vi "Manual with gyro correction - fun no timed loop.vi"() -> ()   [LabVIEW 2017]
panel:
  in  "Encoder Scale":dbl=6.55
  out "y out":dbl format="%#.6f"
  out "x out":dbl format="%#.6f"
  out "Rot spd out":dbl
  out "Remaining delay":dbl
  in  "Period":i64=10
  in  "Delay (s)":dbl
  in  "Motor Stop":bool
  in  "Anticlockwise":bool
  in  "Clockwise":bool
  out "Command from keys":T1(ring)
  in  "Right":bool
  in  "Left":bool
  in  "Down":bool
  in  "Up":bool
  in  "Rot spd multiplier":dbl=2.0
  out "motor 2 out":dbl format="%#.4f"
  out "motor 4 out":dbl format="%#.4f"
  out "motor 3 out":dbl format="%#.4f"
  out "motor 1 out":dbl format="%#.4f"
  out "error out":errorcluster
  in  "error in":errorcluster
  in  "Trans speed":dbl=3.0
  out "Speed C0":T2(graph)
  out "Counter C0":i32
  out "dx/dt C0":dbl
  out "Speed A":T2(graph)
  out "Counter B":i32
  out "Speed B":T2(graph)
  out "dx/dt B":dbl
  out "dt out (s)":dbl format="%.3f"
  in  "PID gains":T3={"proportional gain (Kc)"=0.015, "integral time (Ti, min)"=0.003, "derivative time (Td, min)"=0.0} {"derivative time (Td, min)" format="%.6f"; "integral time (Ti, min)" format="%.6f"; "proportional gain (Kc)" format="%.6f"}
  in  "stop":bool
  out "dx/dt A":dbl
  out "Counter A":i32
  # "P:  Higher the number, higher the abrupt change\nI: Higher the number, the less it tries to overshoot"
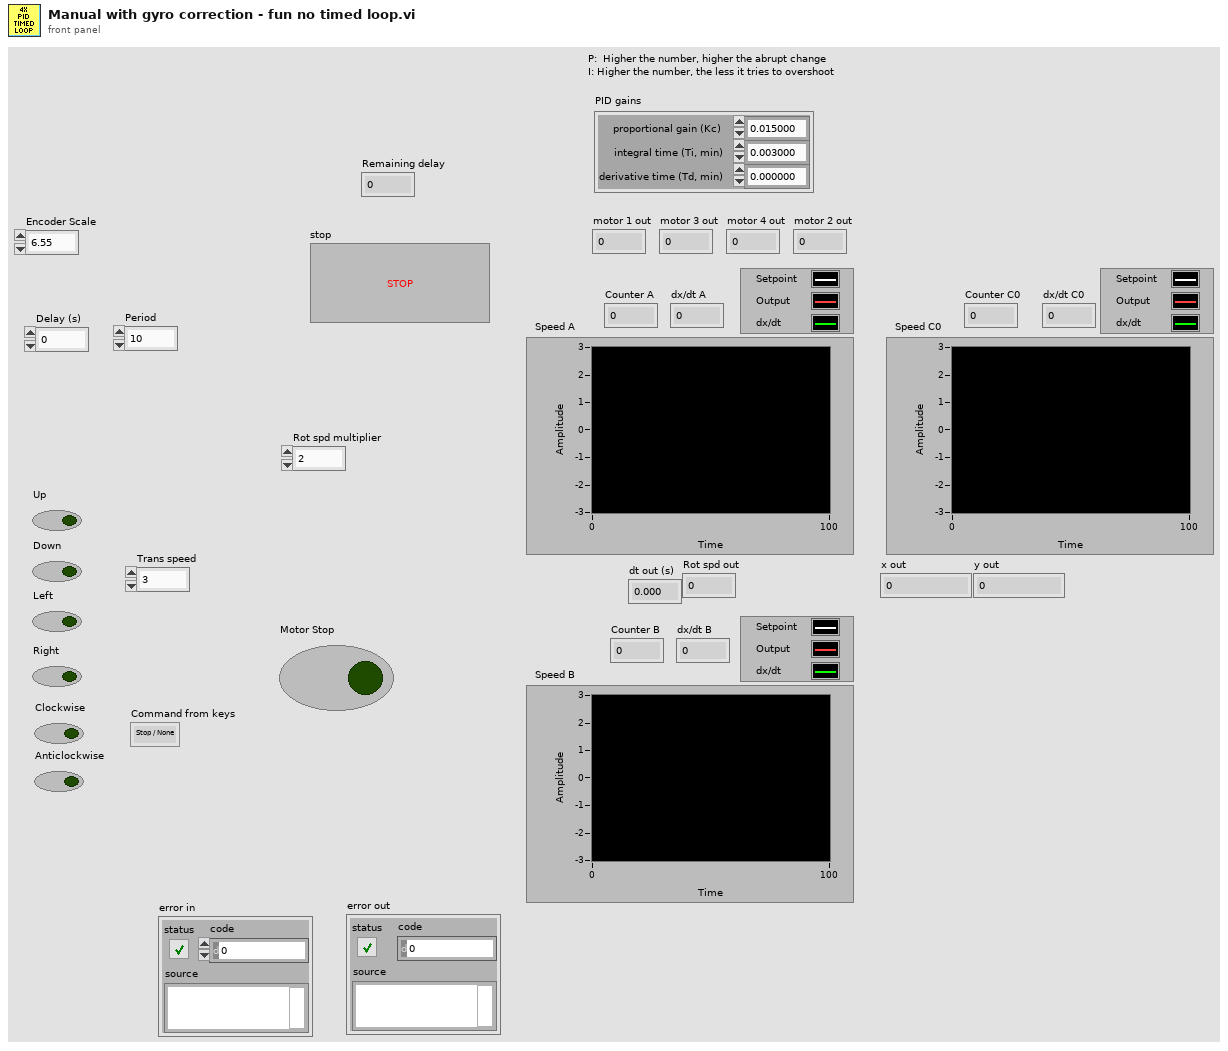
[diagram p1: front panel]
types:
  T1 = enum16{"Stop / None", "Forward", "Backward", "Left", "Right", "Manual"}
  T2 = cluster{"Setpoint":dbl, "output":dbl, "dx/dt":dbl}
  T3 = cluster{"proportional gain (Kc)":dbl, "integral time (Ti, min)":dbl, "derivative time (Td, min)":dbl}
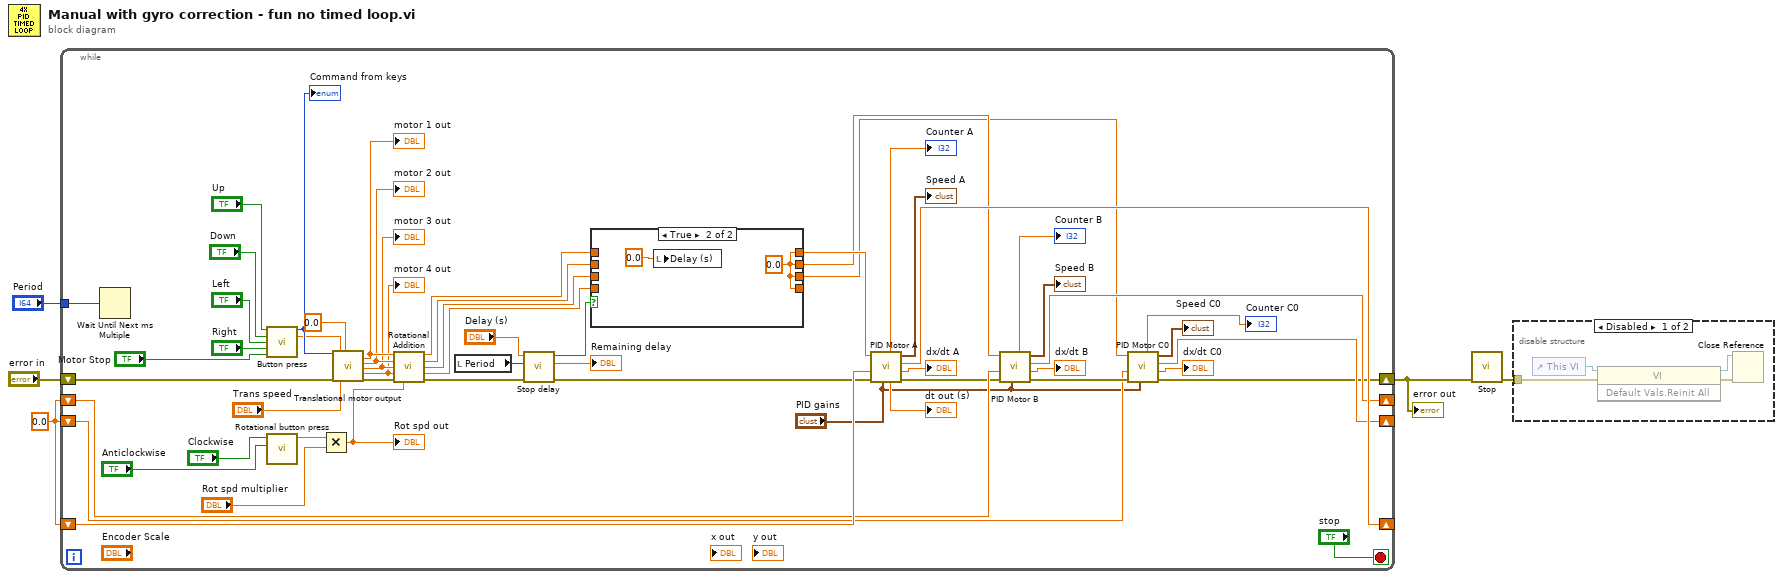
[diagram p0: block diagram]
diagram:
  w5 = 0.0 ("output")
  n1 = while {
    shift-right: [w56] -> _
    shift-left: w5 -> [w60]
    shift-right: [w55] -> _
    shift-left: w5 -> [w54]
    shift-right: [w51] -> _
    shift-left: w5 -> [w50]
    shift-right: [w6] -> w2
    shift-left: "error in" -> [w29]
    tunnel: "Period" -> [w13]
    stop <- "stop" stop-if-true
    n2 = Wait Until Next ms Multiple(millisecond multiple=w13) -> ()  [unwired: 1 out]
    n3 = call "Button press.vi"("Up"="Up", "Down"="Down", "Left"="Left", "Right"="Right", "Stop"="Motor Stop") -> ("Command"=w37:T1, "angle"=w31:dbl)  [unwired: 9 in]
    "Command from keys" <- w37
    n4 = call "Rotational button press.vi"("Anticlockwise"="Anticlockwise", "Clockwise"="Clockwise") -> ("rotDirection"=w7:dbl)  [unwired: 9 in]
    n5 = Multiply(x=w7, y="Rot spd multiplier") -> (x*y=w28:dbl)
    "Rot spd out" <- w28
    n6 = call "Translational motor output.vi"("Command"=w37, "error in"=w29, "manual input angle"=w31, "Trans spd multiplier"="Trans speed", "Orientation"=0.0 ("integral processed")) -> ("motor 1 out"=w43:dbl, "motor 2 out"=w42:dbl, "motor 3 out"=w41:dbl, "motor 4 out"=w40:dbl, "error out"=w39:errorcluster)  [unwired: 10 in]
    "motor 1 out" <- w43
    "motor 3 out" <- w41
    "motor 4 out" <- w40
    "motor 2 out" <- w42
    n7 = call "Rotational Addition.vi"("Motor 1 in"=w43, "Motor 2 in"=w42, "Motor 3 in"=w41, "Motor 4 in"=w40, "error in"=w39, "Rot spd multiplier"=w28) -> ("Motor 1 out"=w27:dbl, "Motor 2 out"=w25:dbl, "Motor 3 out"=w23:dbl, "Motor 4 out"=w21:dbl, "error out"=w20:errorcluster)  [unwired: 5 in]
    n8 = local read "Period"() -> (w16:i64)
    n9 = call "Stop delay.vi"("error in (no error)"=w20, "Period (ms)"=w16, "Delay (s)"="Delay (s)") -> ("error out"=w19:errorcluster, "Remaining delay"=→"Remaining delay":dbl, "Stop?"=w18:bool)  [unwired: 6 in]
    n10 = case shown="True" w18 {
      tunnel: w27 -> [w61 _]
      tunnel: [w61 w66] -> w26
      tunnel: w25 -> [w64 _]
      tunnel: [w64 w66] -> w24
      tunnel: w23 -> [w63 _]
      tunnel: [w63 w66] -> w22
      tunnel: w21 -> [w62 _]
      tunnel: [w62 w66] -> _
      frame False {
      }
      frame True {
        w66 = 0.0 ("Motor 4 out")
        n11 = local write "Delay (s)"(0.0 ("Delay (s)")) -> ()
      }
    }
    n12 = call "PID Motor A.vi"("PID gains"="PID gains", "error in (no error)"=w19, "input"=w60, "Setpoint A0"=w26) -> ("error out"=w45:errorcluster, "dx/dt processed"=→"dx/dt A":dbl, "output"=w56:dbl, "Speed A0"=→"Speed A":T2, "dt out (s)"=→"dt out (s)":dbl, "Counter A0"=→"Counter A":dbl)  [unwired: 2 in]
    n13 = call "PID Motor B.vi"("PID gains"="PID gains", "error in (no error)"=w45, "input"=w54, "Setpoint B0"=w24) -> ("error out"=w52:errorcluster, "dx/dt"=→"dx/dt B":dbl, "output"=w55:dbl, "Speed B0"=→"Speed B":T2, "Counter B0"=→"Counter B":dbl)  [unwired: 2 in, 1 out]
    n14 = call "PID Motor C0.vi"("PID gains"="PID gains", "error in (no error)"=w52, "input"=w50, "Setpoint C0"=w22) -> ("error out"=w6:errorcluster, "dx/dt"=→"dx/dt C0":dbl, "output"=w51:dbl, "Speed C0"=→"Speed C0":T2, "Counter C0"=→"Counter C0":dbl)  [unwired: 2 in, 1 out]
  }
  "error out" <- w2
  n15 = call "Stop.vi"("error in (no error)"=w2) -> ("OG error out"=w3:errorcluster)  [unwired: 9 in, 1 out]
  n16 = disable-structure shown="Disabled" {
    disable-tunnel: w3 -> [w70 _]
    frame Disabled {
      n17 = control-ref of="This VI"() -> (w69:refnum<vi>)
      n18 = invoke class="VI" method="Default Vals.Reinit All"(reference=w69, error in=w70) -> (reference out=w68:refnum<vi>, error out=w67:errorcluster)  [unwired: 1 in, 1 out]
      n19 = Close Reference(reference=w68, error in (no error)=w67) -> ()  [unwired: 1 out]
    }
    frame Enabled {
    }
  }
